vi "断电保存全局.vi"() -> ()   [LabVIEW 2016, in "Alarm interface.lvlib"]
uses:
  Alarm interface.lvlib
panel:
  in  "选项卡控件":enum32{"一级报警", "二级报警", "三级报警"}(tab)
  in  "一级报警":string[][](table)
  in  "二级报警":string[][](table)
  in  "三级报警":string[][](table)
  in  "短信语音用户列表":string[][](array[string])
  in  "报警定义表":string[][](array[string])=[["一级", "短信 电话 微信", "0-1000"], ["二级", "短信 电话 微信", "1001-2000"], ["三级", "短信 电话 微信", "2001-3000"]]
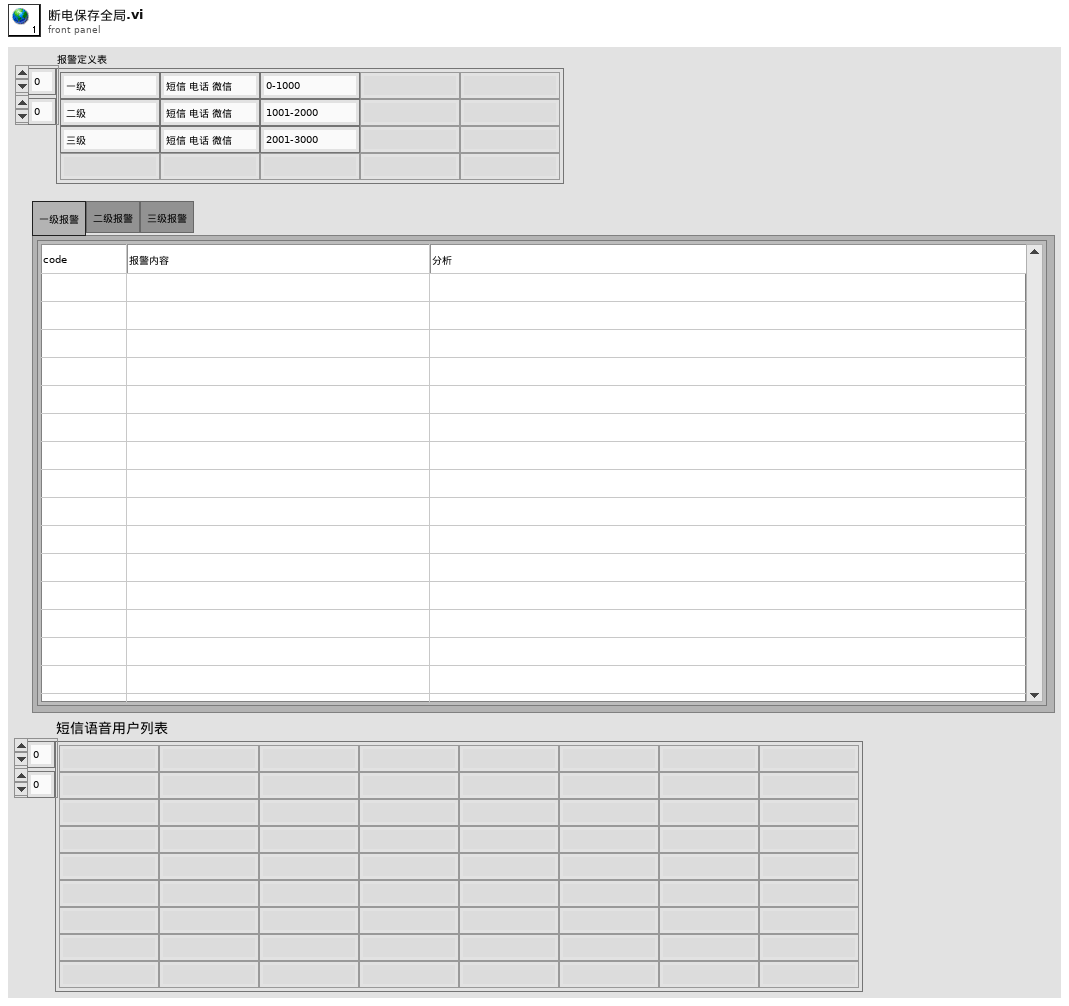
[diagram p1: front panel]
diagram:
